vi "TVEFeRFePlot.vi"(7 "PlotSource":T5, 8 "error in (no error)":errorcluster, 11 "ResultArray":T1 {"Time Stamp" format="%^<%.3X\n%x>T"}) -> (0 "error out":errorcluster, 2 "TVE Fe RFe Plot":T4(graph))   [LabVIEW 2014]
uses:
  typedefs/PlotSource.ctl
  typedefs/ResultArray.ctl
  typedefs/Result.ctl
  typedefs/TVE_Fe_RFE.ctl
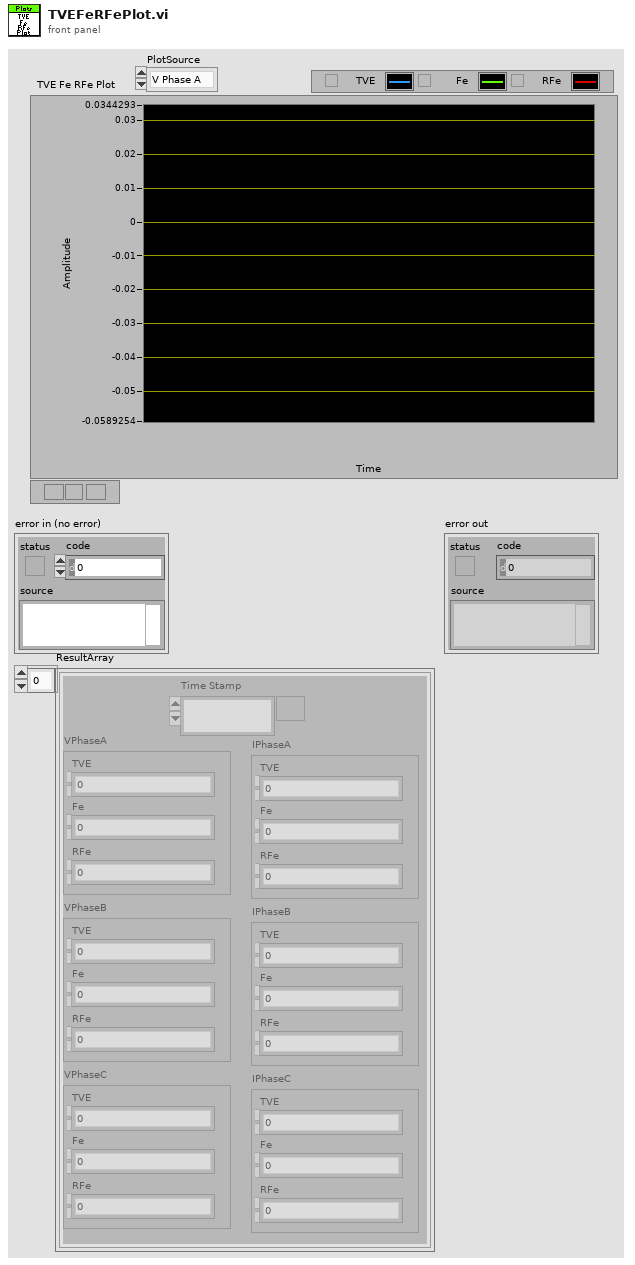
[diagram p1: front panel]
types:
  T1 = typedef "ResultArray.ctl" = T2[]
  T2 = typedef "Result.ctl" = cluster{"Time Stamp":timestamp, "VPhaseA":T3, "VPhaseB":T3, "VPhaseC":T3, "IPhaseA":T3, "IPhaseB":T3, "IPhaseC":T3}
  T3 = typedef "TVE_Fe_RFE.ctl" = cluster{"TVE":dbl, "Fe":dbl, "RFe":dbl}
  T4 = cluster{"TimestampArray":timestamp[], "Y":dbl[]}[]
  T5 = typedef "PlotSource.ctl" = enum16{"V Phase A", "V Phase B", "V Phase C", "I Phase A", "I Phase B", "I Phase C"}
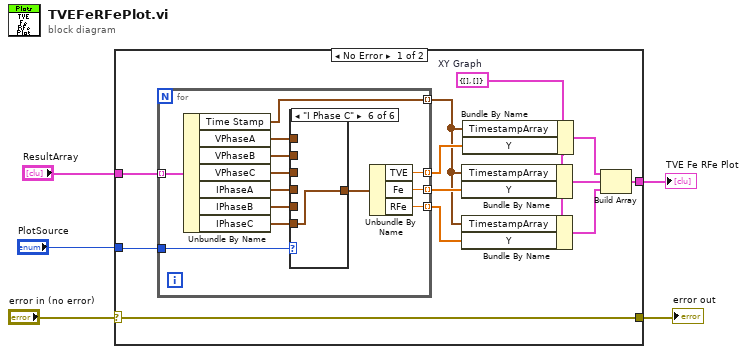
[diagram p0: block diagram]
diagram:
  n1 = case shown="No Error" "error in (no error)" {
    selector: "error in (no error)" -> [w6 w37]
    tunnel: [w6 w37] -> w4
    tunnel: "PlotSource" -> [w16 _]
    tunnel: "ResultArray" -> [w17 _]
    tunnel: [w7 _] -> w1
    frame No Error {
      w15 = cluster{"TimestampArray":timestamp[], "Y":dbl[]} {"TimestampArray"=[], "Y"=[]}  # XY Graph
      n2 = for {
        tunnel: w17 -> [w30] mode=indexing
        tunnel: [w29] -> w11 mode=indexing
        tunnel: w16 -> [w22]
        tunnel: [w20] -> w14 mode=indexing
        tunnel: [w19] -> w13 mode=indexing
        tunnel: [w18] -> w12 mode=indexing
        n3 = Unbundle By Name(w30) -> ("Time Stamp"=w29:timestamp, "VPhaseA"=w28:T3, "VPhaseB"=w27:T3, "VPhaseC"=w26:T3, "IPhaseA"=w25:T3, "IPhaseB"=w24:T3, "IPhaseC"=w23:T3)
        n4 = case shown="\"I Phase C\"" w22 {
          tunnel: w28 -> [w31 _ _ _ _ _]
          tunnel: w27 -> [_ w32 _ _ _ _]
          tunnel: w26 -> [_ _ w33 _ _ _]
          tunnel: w25 -> [_ _ _ w34 _ _]
          tunnel: w24 -> [_ _ _ _ w35 _]
          tunnel: w23 -> [_ _ _ _ _ w36]
          tunnel: [w31 w32 w33 w34 w35 w36] -> w21
          frame "V Phase A", Default {
          }
          frame "V Phase B" {
          }
          frame "V Phase C" {
          }
          frame "I Phase A" {
          }
          frame "I Phase B" {
          }
          frame "I Phase C" {
          }
        }
        n5 = Unbundle By Name(w21) -> ("TVE"=w20:dbl, "Fe"=w19:dbl, "RFe"=w18:dbl)
      }
      n6 = Bundle By Name(cluster=w15, "TimestampArray"=w11, "Y"=w13) -> (w10:cluster{"TimestampArray":timestamp[], "Y":dbl[]})
      n7 = Bundle By Name(cluster=w15, "TimestampArray"=w11, "Y"=w12) -> (w8:cluster{"TimestampArray":timestamp[], "Y":dbl[]})
      n8 = Bundle By Name(cluster=w15, "TimestampArray"=w11, "Y"=w14) -> (w9:cluster{"TimestampArray":timestamp[], "Y":dbl[]})
      n9 = Build Array(w9, w10, w8) -> (w7:T4)
    }
    frame Error {
    }
  }
  "error out" <- w4
  "TVE Fe RFe Plot" <- w1
